vi "keywords enum to array.vi"() -> (2 "enums":T1[](array[typedef]), 3 "strings":string[](array[string]))   [LabVIEW 2024, in "controls manager.lvlib"]
uses:
  controls manager.lvlib
  keywords.ctl
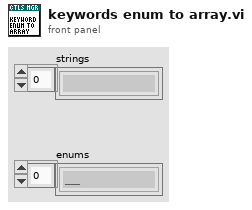
[diagram p1: front panel]
types:
  T1 = typedef "controls manager.lvlib/keywords.ctl" = enum16{"___", "enable", "disable", "gray", "visible", "hidden", "tip", "caption", "blinking", "not_blinking", "page", "default"}
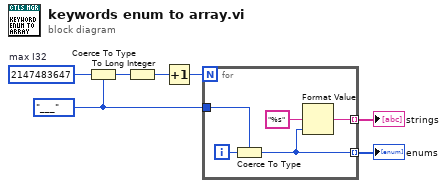
[diagram p0: block diagram]
diagram:
  w3 = 2147483647  # max I32
  w7 = keywords."___"
  n1 = Coerce To Type(0:w3, 1:w7) -> (2:w4:T1)
  n2 = To Long Integer(number=w4) -> (32bit integer=w5:i32)
  n3 = Increment(x=w5) -> (x+1=w6:i32)
  n4 = for {
    N: w6 -> [_]
    tunnel: w7 -> [w11]
    tunnel: [w9] -> w1 mode=indexing
    tunnel: [w8] -> w2 mode=indexing
    i -> [w12]
    n5 = Coerce To Type(0:w12, 1:w11) -> (2:w9:T1)
    n6 = Format Value(format string="%s", value (0)=w9) -> (output string=w8:string)  [unwired: 1 in]
  }
  "strings" <- w2
  "enums" <- w1
